vi "Close.vi"(8 "error in (no error)":errorcluster, 11 "VICI Settings":T1) -> (0 "error out":errorcluster, 1 "Connection Error":bool, 3 "VICI Settings":T1)   [LabVIEW 2018, in "VICI M6 M50 Party Mode.lvlib"]
uses:
  VICI M6 M50 Party Mode.lvlib
  Settings Cluster.ctl
  VICI Global Library.lvlib
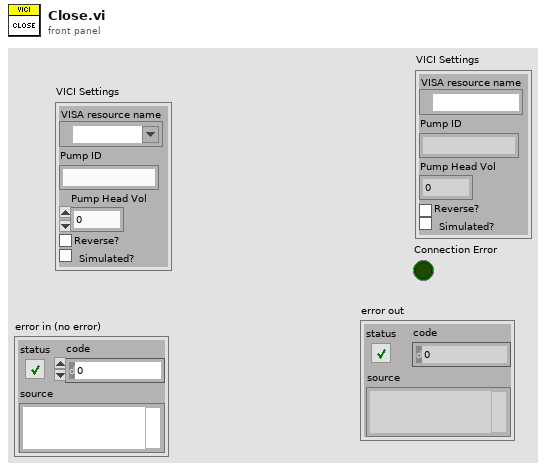
[diagram p1: front panel]
types:
  T1 = typedef "VICI M6 M50 Party Mode.lvlib/Settings Cluster.ctl" = cluster{"VISA resource name":refnum<visa-resource-name>, "Pump ID":string, "Pump Head Vol":dbl, "Reverse?":bool, "Simulated?":bool}
  T2 = typedef "VICI M6 M50 Party Mode.lvlib/VICI Global Library.lvlib/VICI Global.ctl" = cluster{"Busy":bool, "VISA #":string, "Current Pump":string, "Current Function":string, "Pump Array":string[], "Last Success":timestamp, "ID Queue":string[]}
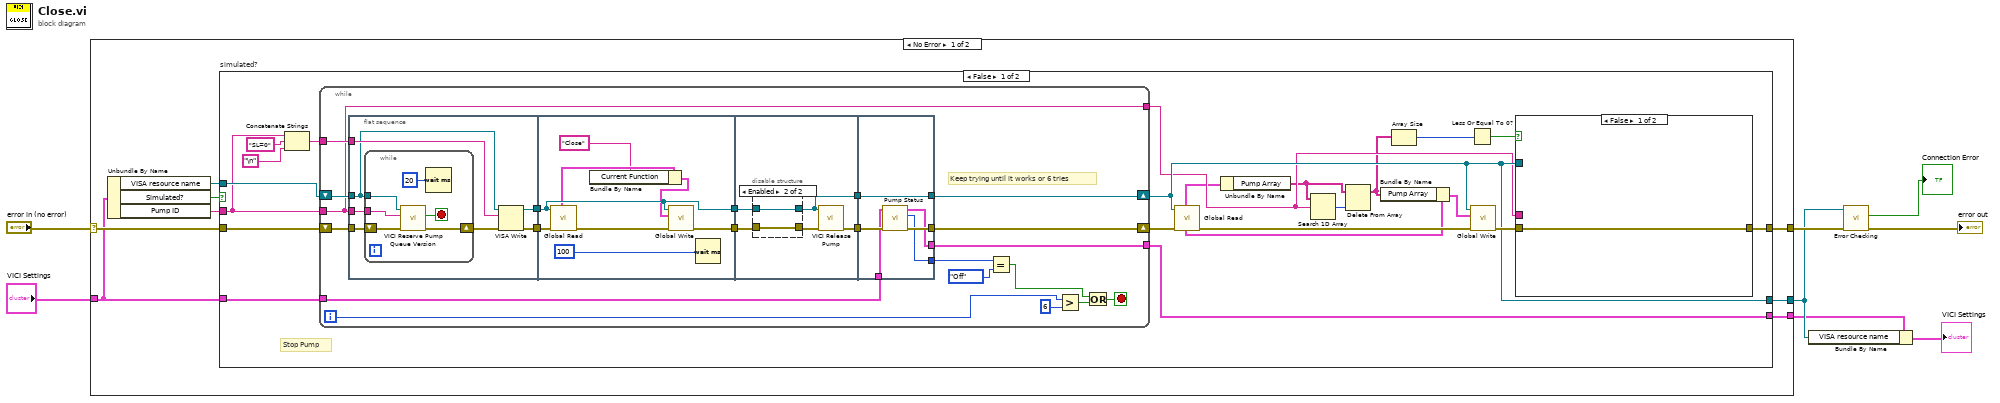
[diagram p0: block diagram]
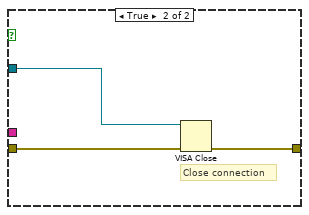
[diagram p2: hidden frame]
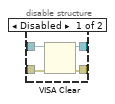
[diagram p3: hidden frame]
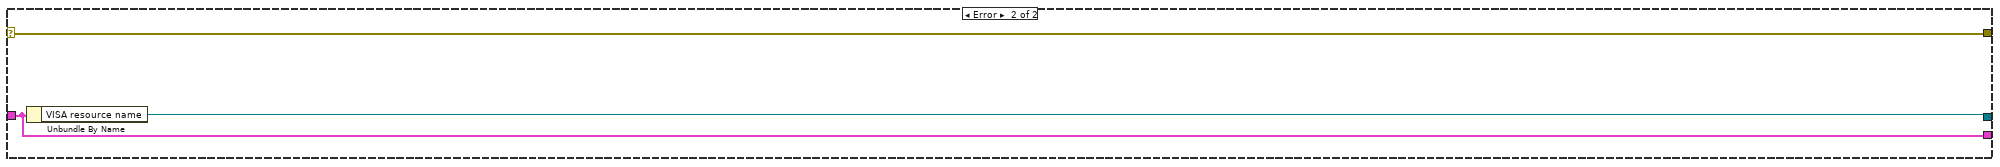
[diagram p5: hidden frame]
diagram:
  n1 = case shown="No Error" "error in (no error)" {
    selector: "error in (no error)" -> [w14 w106]
    tunnel: [w15 w106] -> w6
    tunnel: "VICI Settings" -> [w11 w104]
    tunnel: [w12 w105] -> w3
    tunnel: [w10 w104] -> w2
    frame No Error {
      n2 = Unbundle By Name(w11) -> ("VISA resource name"=w13:refnum<visa-resource-name>, "Simulated?"=w16:bool, "Pump ID"=w9:string)
      n3 = case "simulated?" shown="False" w16 {
        tunnel: [w29 w103] -> w15
        tunnel: w13 -> [w33 w102]
        tunnel: w14 -> [w35 w103]
        tunnel: [w25 w102] -> w12
        tunnel: w11 -> [w32 w101]
        tunnel: [w31 w101] -> w10
        tunnel: w9 -> [w30 _]
        frame False {
          # "Stop Pump"
          n4 = Concatenate Strings(w30, "SL=0" ("string"), "\n") -> (w34:string)
          n5 = while {
            tunnel: w34 -> [w55]
            shift-right: [w54] -> w28
            shift-left: w35 -> [w56]
            shift-right: [w52] -> w25
            shift-left: w33 -> [w53]
            tunnel: w32 -> [w51]
            tunnel: [w50] -> w31
            tunnel: w30 -> [w47]
            tunnel: [w47] -> w24
            i -> [w44]
            stop <- w42 stop-if-true
            # "Keep trying until it works or 6 tries"
            n6 = flat-sequence {
              tunnel: [w67] -> w62
              tunnel: [w68] -> w61
              tunnel: w56 -> [w66]
              tunnel: w55 -> [w69]
              tunnel: w53 -> [w64]
              tunnel: w47 -> [w63]
              tunnel: w62 -> [w79]
              tunnel: [w79] -> w60
              tunnel: w61 -> [w82]
              tunnel: [w80] -> w59
              tunnel: w60 -> [w88]
              tunnel: w59 -> [w87]
              tunnel: [w84] -> w58
              tunnel: [w86] -> w57
              tunnel: [w100] -> w52
              tunnel: [w98] -> w54
              tunnel: w58 -> [w99]
              tunnel: w57 -> [w100]
              tunnel: [w97] -> w49
              tunnel: w51 -> [w96]
              tunnel: [w95] -> w50
              frame #0 {
                n7 = while {
                  tunnel: w64 -> [w74]
                  tunnel: w63 -> [w73]
                  shift-right: [w70] -> w65
                  shift-left: w66 -> [w72]
                  stop <- w71 stop-if-true
                  n8 = call "VICI Reserve Pump Queue Version.vi"("error in (no error)"=w72, "Pump ID"=w73, "VISA # in"=w74) -> ("error out"=w70:errorcluster, "Loop Completed"=w71:bool)  [unwired: 6 in, 1 out]
                  n9 = Wait (ms)(milliseconds to wait=u32 20) -> ()  [unwired: 1 out]
                }
                n10 = VISA Write(VISA resource name=w64, write buffer=w69, error in (no error)=w65) -> (VISA resource name out=w67:refnum<visa-resource-name>, error out=w68:errorcluster)  [unwired: 1 out]
              }
              frame #1 {
                n11 = call "Global Read.vi"("VISA #"=w79, "error in (no error)"=w82) -> ("Global for this VISA"=w78:T2, "error out"=w81:errorcluster)  [unwired: 2 in, 5 out]
                n12 = Bundle By Name(cluster=w78, "Current Function"="Close") -> (w77:T2)
                n13 = call "Global Write.vi"("error in (no error)"=w81, "VICI Global"=w77, "VISA # in"=w79) -> ("error out"=w80:errorcluster)  [unwired: 7 in, 1 out]
                n14 = Wait (ms)(milliseconds to wait=u32 100) -> ()  [unwired: 1 out]
              }
              frame #2 {
                n15 = disable-structure shown="Enabled" {
                  disable-tunnel: w88 -> [w92 w94]
                  disable-tunnel: w87 -> [w91 w93]
                  disable-tunnel: [w90 w94] -> w86
                  disable-tunnel: [w89 w93] -> w85
                  frame Disabled {
                    n16 = VISA Clear(VISA resource name=w92, error in (no error)=w91) -> (VISA resource name out=w90:refnum<visa-resource-name>, error out=w89:errorcluster)
                  }
                  frame Enabled {
                  }
                }
                n17 = call "VICI Release Pump.vi"("error in (no error)"=w85, "VISA # in"=w86) -> ("error out"=w84:errorcluster)  [unwired: 8 in, 1 out]
              }
              frame #3 {
                n18 = call "Pump Status.vi"("error in (no error)"=w99, "VICI Settings In"=w96) -> ("error out"=w98:errorcluster, "Pump On?"=w97:enum16{"Off", "On", "Not Initialized"}, "VICI Settings Out"=w95:T1)  [unwired: 6 in, 1 out]
              }
            }
            n19 = Equal?(x=w49, y=enum16{"Off", "On", "Not Initialized"}."Off") -> (x = y?=w43:bool)
            n20 = Greater?(x=w44, y=6) -> (0:w45:bool)
            n21 = Or(x=w43, y=w45) -> (x .or. y?=w42:bool)
          }
          n22 = call "Global Read.vi"("VISA #"=w25, "error in (no error)"=w28) -> ("Global for this VISA"=w21:T2, "error out"=w27:errorcluster)  [unwired: 2 in, 5 out]
          n23 = Unbundle By Name(w21) -> ("Pump Array"=w22:string[])
          n24 = Search 1D Array(1D array=w22, element=w24) -> (index of element=w23:i32)  [unwired: 1 in]
          n25 = Delete From Array(array=w22, index=w23) -> (array with subset deleted=w19:string[])  [unwired: 1 in, 1 out]
          n26 = Bundle By Name(cluster=w21, "Pump Array"=w19) -> (w20:T2)
          n27 = Array Size(array=w19) -> (size(s)=w18:i32)
          n28 = Less Or Equal To 0?(x=w18) -> (x <= 0?=w17:bool)
          n29 = call "Global Write.vi"("error in (no error)"=w27, "VICI Global"=w20, "VISA # in"=w25) -> ("error out"=w26:errorcluster)  [unwired: 7 in, 1 out]
          n30 = case shown="False" w17 {
            tunnel: [w38 w41] -> w29
            tunnel: w26 -> [w38 w40]
            tunnel: w25 -> [_ w39]
            tunnel: w24 -> [_ _]
            frame False {
            }
            frame True {
              # "Close connection"
              n31 = VISA Close(VISA resource name=w39, error in (no error)=w40) -> (error out=w41:errorcluster)
            }
          }
        }
        frame True {
        }
      }
    }
    frame Error {
      n32 = Unbundle By Name(w104) -> ("VISA resource name"=w105:refnum<visa-resource-name>)
    }
  }
  n33 = Bundle By Name(cluster=w2, "VISA resource name"=w3) -> (→"VICI Settings":T1)
  n34 = call "Error Checking.vi"("error in (no error)"=w6, "VISA resource name"=w3) -> ("error out"=→"error out":errorcluster, "Connection Error"=→"Connection Error":bool)  [unwired: 7 in, 1 out]
